vi "DQMH System Message - Removed from Subpanel.vi"(11 "Removed Module":string) -> (1 "Payload":variant, 2 "Identifier":string="Removed from Subpanel", 5 "Source":T1)   [LabVIEW 2020, in "hse-dqmh.lvlib"]
doc: "____\nHAMPEL SOFTWARE ENGINEERING v3.8.0 (2023-12-18 14:41)"
uses:
  hse-dqmh.lvlib
  Controls/System Message Source.ctl
  Controls/System Message Framework Identifiers.ctl
  Controls/System Message - Removed from Subpanel - Payload--cluster.ctl
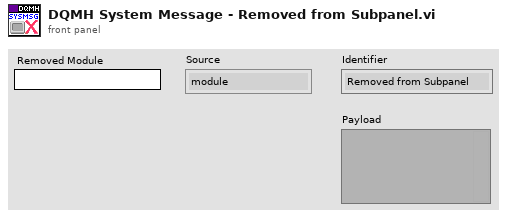
[diagram p1: front panel]
types:
  T1 = typedef "hse-dqmh.lvlib/System Message Source.ctl" = enum16{"module", "application", "network"}
  T2 = typedef "hse-dqmh.lvlib/System Message - Removed from Subpanel - Payload--cluster.ctl" = cluster{"Removed Module":string}
  T3 = typedef "hse-dqmh.lvlib/System Message Framework Identifiers.ctl" = enum16{"Add to Run-Time Menu", "Ready for Display", "Removed from Subpanel", "Remove from Run-Time Menu"}
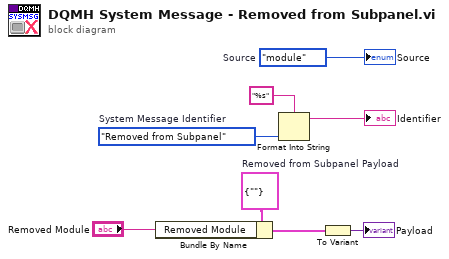
[diagram p0: block diagram]
diagram:
  w3 = T2 {"Removed Module"=""}  # Removed from Subpanel Payload
  w6 = System_Message_Framework_Identifiers."Removed from Subpanel"  # System Message Identifier
  w8 = System_Message_Source."module"  # Source
  n1 = Bundle By Name(cluster=w3, "Removed Module"="Removed Module") -> (w2:T2)
  n2 = Format Into String(format string="%s", w6) -> (resulting string=→"Identifier":string)  [unwired: 2 in, 1 out]
  n3 = To Variant(anything=w2) -> (Variant=→"Payload":variant)
  "Source" <- w8
